vi "Command Callback.vi"(11 "Timer ID":u8) -> ()   [LabVIEW 2015]
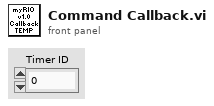
[diagram p1: front panel]
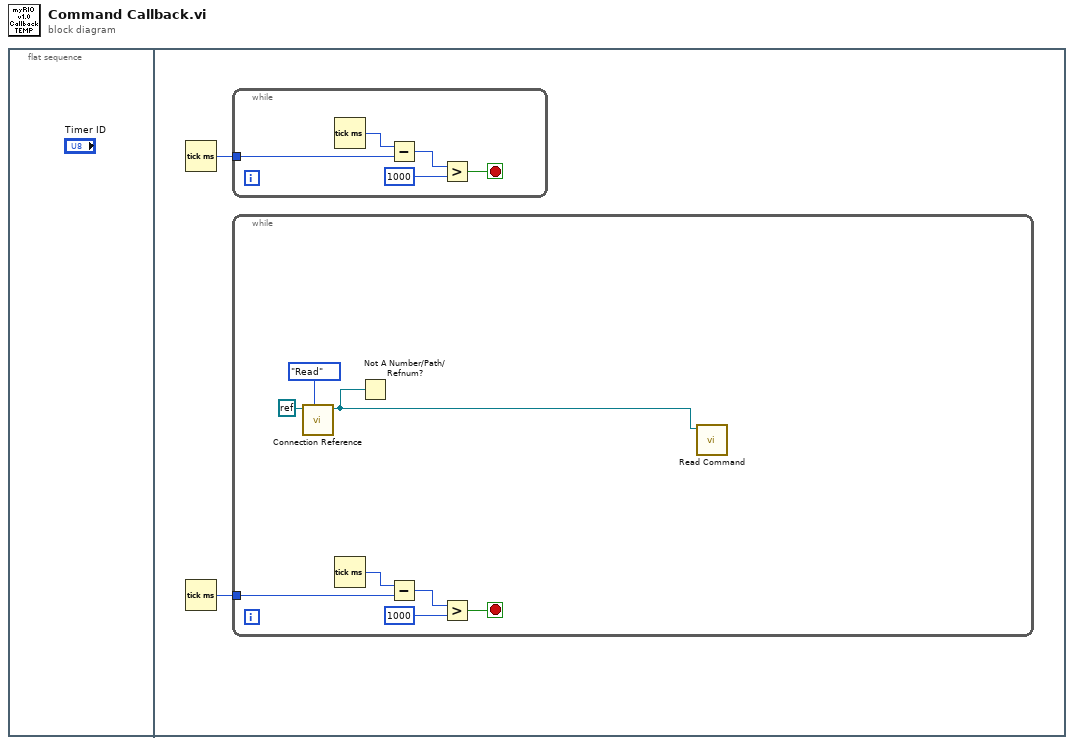
[diagram p0: block diagram]
diagram:
  n1 = flat-sequence {
    frame #0 {
    }
    frame #1 {
      n2 = Tick Count (ms)() -> (millisecond timer value=w2:u32)
      n3 = Tick Count (ms)() -> (millisecond timer value=w1:u32)
      n4 = while {
        tunnel: w2 -> [w12]
        stop <- w11 stop-if-true
        n5 = Tick Count (ms)() -> (millisecond timer value=w13:u32)
        n6 = Subtract(x=w13, y=w12) -> (x-y=w14:u32)
        n7 = Greater?(x=w14, y=u32 1000) -> (0:w11:bool)
      }
      n8 = while {
        tunnel: w1 -> [w7]
        stop <- w6 stop-if-true
        n9 = call "Connection Reference.vi"("action"=enum16{"Write", "Read"}."Read", "connection ID in"=refnum<k0> refnum) -> ("connection ID out"=w4:refnum<k5>)  [unwired: 9 in]
        n10 = Tick Count (ms)() -> (millisecond timer value=w8:u32)
        n11 = Not A Number/Path/Refnum?(number/path/refnum=w4) -> ()  [unwired: 1 out]
        n12 = Subtract(x=w8, y=w7) -> (x-y=w9:u32)
        n13 = Greater?(x=w9, y=u32 1000) -> (0:w6:bool)
        n14 = call "Read Command.vi"("Connection ID in"=w4) -> ()  [unwired: 9 in, 2 out]
      }
    }
  }
